vi "send_samples.vi"(2 "error in (no error)":errorcluster, 3 "VISA Refnum in":refnum<visa-resource-name>, 4 "elemszam":u8, 5 "periods":u8=1) -> (0 "error out":errorcluster, 1 "VISA Refnum out":refnum<visa-resource-name>)   [LabVIEW 2014]
uses:
  <vilib>/Analysis/NI_AALBase.lvlib
panel:
  out "need to run":bool
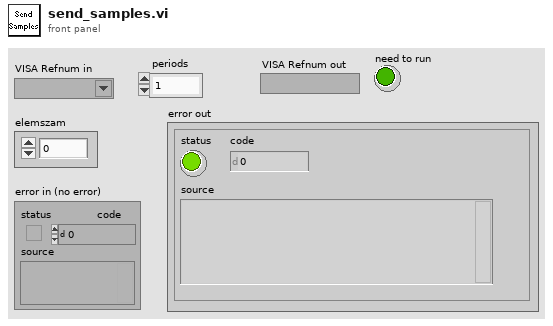
[diagram p1: front panel]
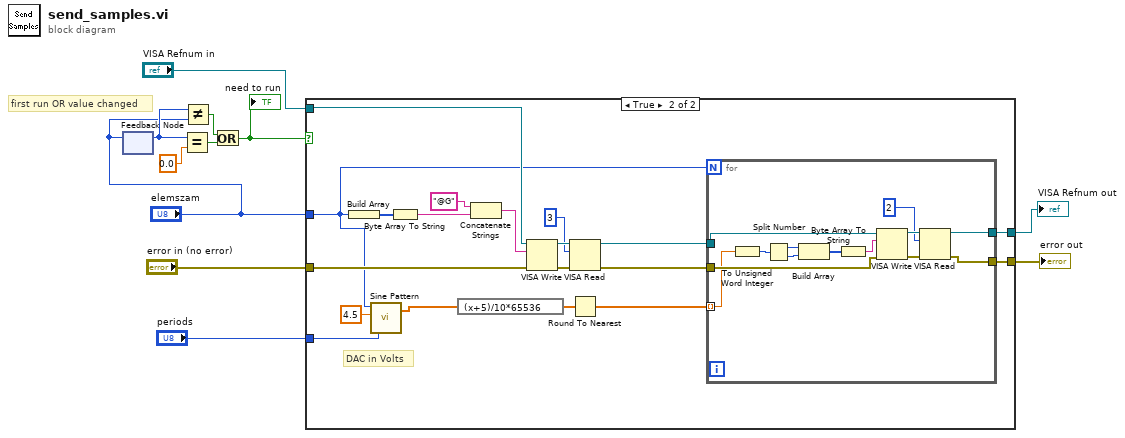
[diagram p0: block diagram]
diagram:
  # "first run OR value changed"
  n1 = feedback #1() -> (w6:u8)  [unwired: 1 in]
  n2 = feedback-in #1("elemszam") -> ()
  n3 = Equal?(x=w6, y=0.0) -> (x = y?=w4:bool)
  n4 = Not Equal?(x=w6, y="elemszam") -> (x != y?=w3:bool)
  n5 = Or(x=w3, y=w4) -> (x .or. y?=w1:bool)
  "need to run" <- w1
  n6 = case shown="True" w1 {
    tunnel: [w12 w32] -> w11
    tunnel: [w13 w31] -> w10
    tunnel: "VISA Refnum in" -> [w13 w21]
    tunnel: "error in (no error)" -> [w12 w20]
    tunnel: "periods" -> [_ w15]
    tunnel: "elemszam" -> [_ w14]
    frame False {
    }
    frame True {
      # "DAC in Volts"
      n7 = Build Array(w14) -> (w27:u8[])
      n8 = call <vilib>:"Sine Pattern.vi"("cycles"=w15, "amplitude"=4.5, "samples"=w14) -> ("Sinusoidal Pattern"=w16:dbl[])  [unwired: 1 in, 1 out]
      n9 = Byte Array To String(unsigned byte array=w27) -> (string=w28:string)
      n10 = expression code="(x+5)/10*65536"(w16) -> (w19:dbl[])
      n11 = Concatenate Strings("@G" ("write buffer"), w28) -> (w23:string)
      n12 = VISA Write(VISA resource name=w21, write buffer=w23, error in (no error)=w20) -> (VISA resource name out=w25:refnum<visa-resource-name>, error out=w26:errorcluster)  [unwired: 1 out]
      n13 = VISA Read(VISA resource name=w25, byte count=u32 3, error in (no error)=w26) -> (VISA resource name out=w30:refnum<visa-resource-name>, error out=w29:errorcluster)  [unwired: 2 out]
      n14 = Round To Nearest(number=w19) -> (nearest integer value=w17:dbl[])
      n15 = for {
        N: w14 -> [_]
        tunnel: w17 -> [w38] mode=indexing
        tunnel: w29 -> [w44]
        tunnel: w30 -> [w43]
        tunnel: [w34] -> w31
        tunnel: [w33] -> w32
        n16 = To Unsigned Word Integer(number=w38) -> (unsigned 16bit integer=w41:u16)
        n17 = Split Number(x=w41) -> (hi(x)=w39:u8, lo(x)=w40:u8)
        n18 = Build Array(w39, w40) -> (w42:u8[])
        n19 = Byte Array To String(unsigned byte array=w42) -> (string=w37:string)
        n20 = VISA Write(VISA resource name=w43, write buffer=w37, error in (no error)=w44) -> (VISA resource name out=w36:refnum<visa-resource-name>, error out=w45:errorcluster)  [unwired: 1 out]
        n21 = VISA Read(VISA resource name=w36, byte count=u32 2, error in (no error)=w45) -> (VISA resource name out=w34:refnum<visa-resource-name>, error out=w33:errorcluster)  [unwired: 2 out]
      }
    }
  }
  "VISA Refnum out" <- w10
  "error out" <- w11
